vi "Write Accounts info.vi"(7 "Index of Account":i32, 8 "error in (no error)":errorcluster, 9 "Account Info":T2, 10 "Accounts info in":T1, 11 "Accounts.txt file path":path) -> (0 "error out":errorcluster, 3 "Accounts info out":T1)   [LabVIEW 2020, in "ATM.lvlib"]
doc: "This VI Updates the Account.txt file with the updated client data"
uses:
  ATM.lvlib
  Accounts Info -- cluster.ctl
  Account Info -- cluster.ctl
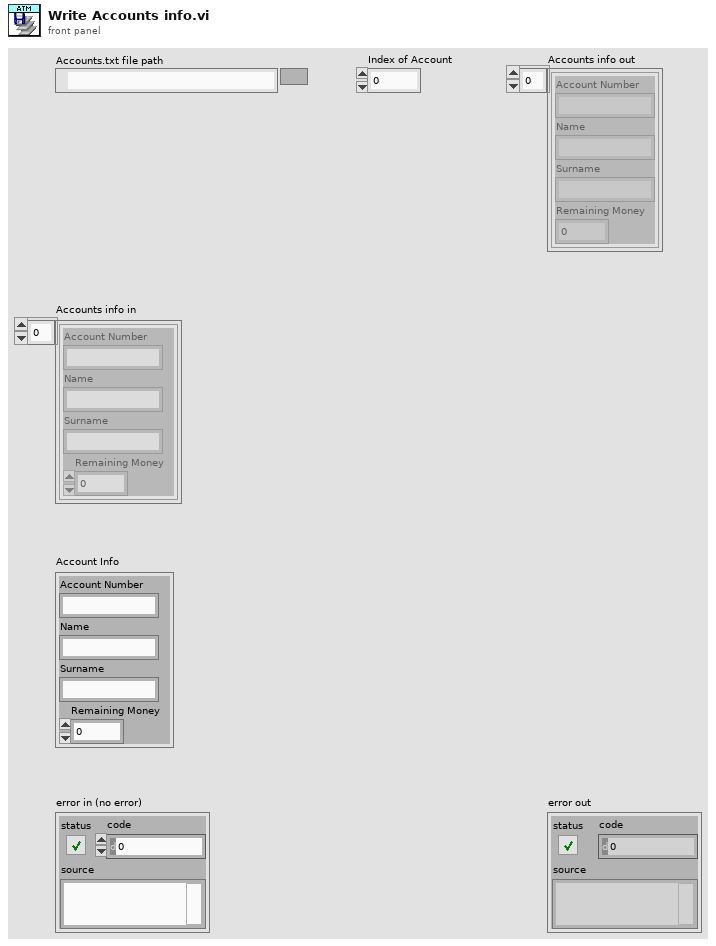
[diagram p1: front panel]
types:
  T1 = typedef "ATM.lvlib/Accounts Info -- cluster.ctl" = T2[]
  T2 = typedef "ATM.lvlib/Account Info -- cluster.ctl" = cluster{"Account Number":string, "Name":string, "Surname":string, "Remaining Money":i32}
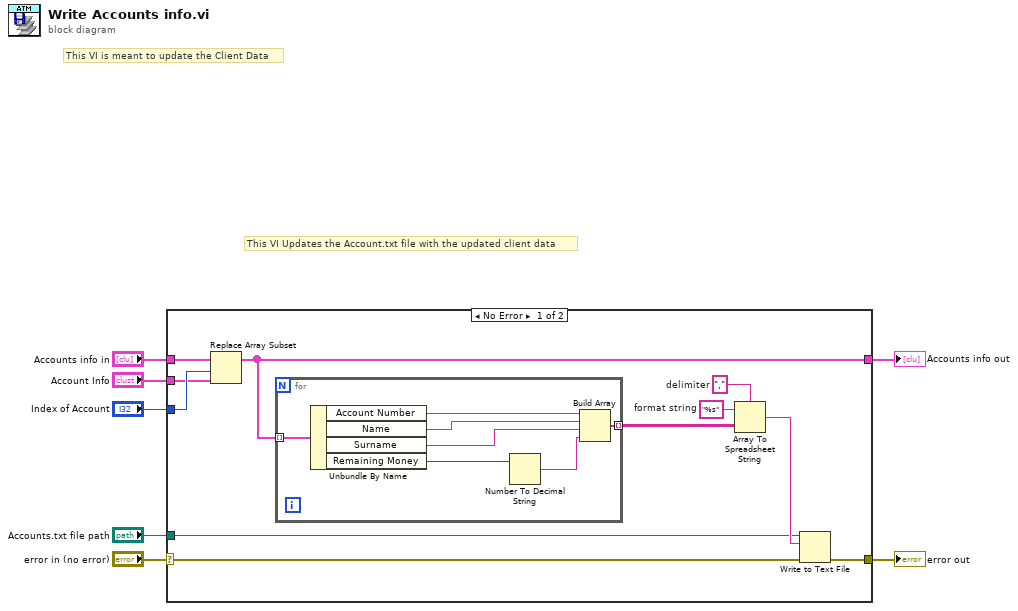
[diagram p0: block diagram]
diagram:
  # "This VI Updates the Account.txt file with the updated client data"
  # "This VI is meant to update the Client Data"
  n1 = case shown="No Error" "error in (no error)" {
    selector: "error in (no error)" -> [w8 w27]
    tunnel: "Accounts info in" -> [w14 w26]
    tunnel: "Index of Account" -> [w13 _]
    tunnel: "Account Info" -> [w12 _]
    tunnel: [w11 w26] -> w4
    tunnel: "Accounts.txt file path" -> [w10 _]
    tunnel: [w9 w27] -> w2
    frame No Error {
      w16 = "%s"  # format string
      w17 = ","  # delimiter
      n2 = Replace Array Subset(array=w14, new element=w12, index=w13) -> (w11:T1)
      n3 = for {
        tunnel: w11 -> [w20] mode=indexing
        tunnel: [w19] -> w15 mode=indexing
        n4 = Unbundle By Name(w20) -> ("Account Number"=w21:string, "Name"=w22:string, "Surname"=w23:string, "Remaining Money"=w24:i32)
        n5 = Number To Decimal String(number=w24) -> (decimal integer string=w25:string)  [unwired: 1 in]
        n6 = Build Array(w21, w22, w23, w25) -> (w19:string[])
      }
      n7 = Array To Spreadsheet String(delimiter (Tab)=w17, array=w15, 3:w16) -> (spreadsheet string=w18:string)
      n8 = Write to Text File(file (use dialog)=w10, text=w18, error in=w8) -> (error out=w9:errorcluster)  [unwired: 1 in, 2 out]
    }
    frame Error {
    }
  }
  "Accounts info out" <- w4
  "error out" <- w2
